vi "sub_ekf_estimation.vi"(8 "z":T1, 9 "ud":T1, 10 "PEst":T1, 11 "xEst":T1) -> (2 "PEst":T1, 3 "xEst":T1)   [LabVIEW 2019]
uses:
  <vilib>/Analysis/Matrix/Datatypes/RealMatrix.ctl
  Ctrl/cmd_common.ctl
  <vilib>/Analysis/Matrix/Numeric/Multiply/Multiply - RM,RM.vi
  <vilib>/Analysis/Matrix/Numeric/Add/Add - RM,RM.vi
  <vilib>/Analysis/Matrix/Numeric/Subtract/Subtract - RM,RM.vi
  <vilib>/Analysis/baseanly.llb/Real Inverse Matrix.vi
  <vilib>/Analysis/Matrix/NI_Matrix.lvlib
  <vilib>/Analysis/NI_AALBase.lvlib
panel:
  out "PPred":T1
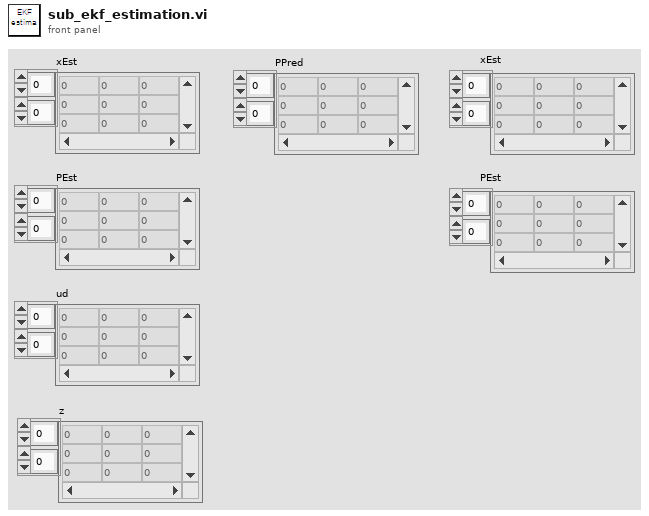
[diagram p1: front panel]
types:
  T1 = typedef "NI_Matrix.lvlib/RealMatrix.ctl" = dbl[][]
  T2 = typedef "cmd_common.ctl" = enum16{"read", "write"}
  T3 = cluster{"Q":T1, "R":T1, "input Noise":T1, "GPS noise":T1, "DT":dbl}
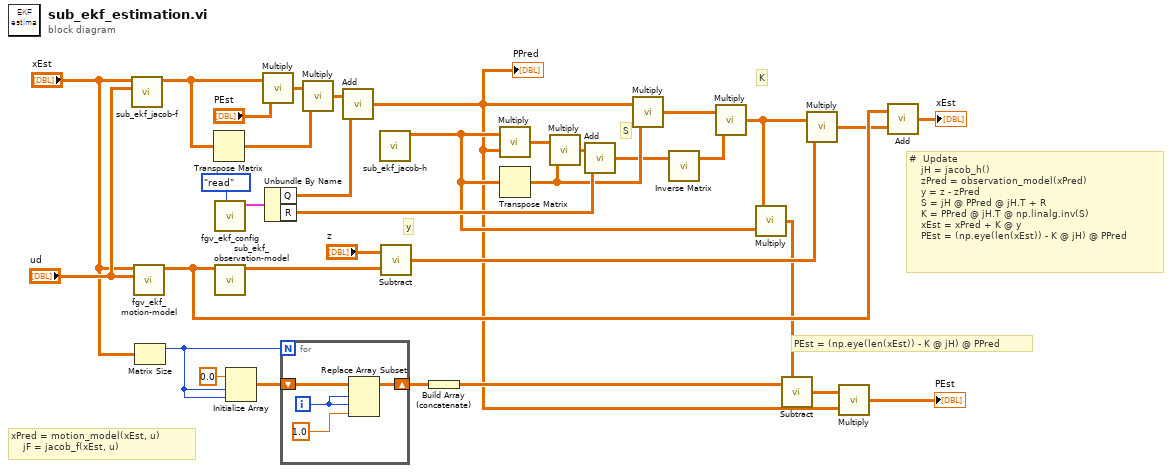
[diagram p0: block diagram]
diagram:
  # "PEst = (np.eye(len(xEst)) - K @ jH) @ PPred"
  # "xPred = motion_model(xEst, u)\n    jF = jacob_f(xEst, u)"
  # "#  Update\n    jH = jacob_h()\n    zPred = observation_model(xPred)\n    y = z - zPred\n    S = jH @ PPred @ jH.T + R\n    K = PPred @ jH.T @ np.linalg.inv(S)\n    xEst = xPred + K @ y\n    PEst = (np.eye(len(xEst)) - K @ jH) @ PPred"
  # "K"
  # "S"
  # "y"
  n1 = call "sub_ekf_jacob-f.vi"("ud"="ud", "xEst"="xEst") -> ("jF"=w30:T1)  [unwired: 9 in]
  n2 = call "fgv_ekf_motion-model.vi"("u"="ud", "x_true"="xEst") -> ("x_true out"=w19:T1)  [unwired: 9 in]
  n3 = Matrix Size(0:"xEst") -> (1:w10:i32)  [unwired: 1 out]
  n4 = Transpose Matrix(1:w30) -> (0:w32:T1)
  n5 = call "fgv_ekf_config.vi"("cmd"=cmd_common."read") -> ("set var out"=w28:T3)  [unwired: 10 in]
  n6 = call "sub_ekf_observation-model.vi"("x_true"=w19) -> ("x_true out"=w24:T1)  [unwired: 10 in]
  n7 = Initialize Array(0.0 ("원소"), w10, w10) -> (w9:dbl[][])
  n8 = call-poly <vilib>:"Multiply.vi"("Real Matrix B"="PEst", "Real Matrix A"=w30) -> ("A * B"=w31:T1)
  n9 = Unbundle By Name(w28) -> ("Q"=w33:T1, "R"=w21:T1)
  n10 = for {
    N: w10 -> [_]
    shift-right: [w35] -> w8
    shift-left: w9 -> [w38]
    i -> [w37]
    n11 = Replace Array Subset(array=w38, new element=1.0 ("새 원소/부분배열"), index (row)=w37, index (col)=w37) -> (w35:dbl[][])
  }
  n12 = call-poly <vilib>:"Multiply.vi"("Real Matrix B"=w32, "Real Matrix A"=w31) -> ("A * B"=w34:T1)
  n13 = call-poly <vilib>:"Add.vi"("Real Matrix B"=w33, "Real Matrix A"=w34) -> ("A + B"=w2:T1)
  "PPred" <- w2
  n14 = call "sub_ekf_jacob-h.vi"() -> ("jH"=w6:T1)  [unwired: 11 in]
  n15 = call-poly <vilib>:"Subtract.vi"("Real Matrix B"=w24, "Real Matrix A"="z") -> ("A - B"=w15:T1)
  n16 = Build Array (concatenate)(w8) -> (w5:T1)
  n17 = call-poly <vilib>:"Multiply.vi"("Real Matrix B"=w2, "Real Matrix A"=w6) -> ("A * B"=w23:T1)
  n18 = Transpose Matrix(1:w6) -> (0:w20:T1)
  n19 = call-poly <vilib>:"Multiply.vi"("Real Matrix B"=w20, "Real Matrix A"=w23) -> ("A * B"=w22:T1)
  n20 = call-poly <vilib>:"Add.vi"("Real Matrix B"=w21, "Real Matrix A"=w22) -> ("A + B"=w18:T1)
  n21 = call-poly <vilib>:"Multiply.vi"("Real Matrix B"=w20, "Real Matrix A"=w2) -> ("A * B"=w17:T1)
  n22 = call-poly <vilib>:"Inverse Matrix.vi"("Input Matrix"=w18) -> ("Inverse Matrix"=w16:T1)  [unwired: 1 in, 1 out]
  n23 = call-poly <vilib>:"Multiply.vi"("Real Matrix B"=w16, "Real Matrix A"=w17) -> ("A * B"=w7:T1)
  n24 = call-poly <vilib>:"Multiply.vi"("Real Matrix B"=w6, "Real Matrix A"=w7) -> ("A * B"=w4:T1)
  n25 = call-poly <vilib>:"Subtract.vi"("Real Matrix B"=w4, "Real Matrix A"=w5) -> ("A - B"=w3:T1)
  n26 = call-poly <vilib>:"Multiply.vi"("Real Matrix B"=w15, "Real Matrix A"=w7) -> ("A * B"=w14:T1)
  n27 = call-poly <vilib>:"Multiply.vi"("Real Matrix B"=w2, "Real Matrix A"=w3) -> ("A * B"=→"PEst":T1)
  n28 = call-poly <vilib>:"Add.vi"("Real Matrix B"=w14, "Real Matrix A"=w19) -> ("A + B"=→"xEst":T1)
